vi "Fade In.vi"(7 "Stop Demo":refnum<user-event>, 8 "error in":errorcluster, 10 "VI":refnum<vi>, 11 "Main Subpanel":refnum<vi>) -> (0 "error out":errorcluster)   [LabVIEW 2020]
uses:
  <vilib>/Utility/miscctls.llb/LVRectTypeDef.ctl
  <vilib>/Utility/miscctls.llb/LVPointTypeDef.ctl
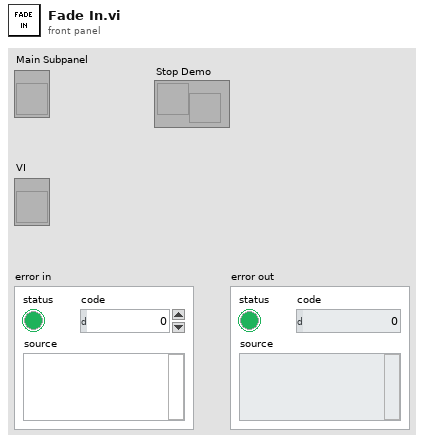
[diagram p1: front panel]
types:
  T1 = typedef "LVPointTypeDef.ctl" = cluster{"Horizontal":i16, "Vertical":i16}
  T2 = enum32{"Invalid", "Standard", "Closed", "Hidden", "Minimized", "Maximized"}
  T3 = typedef "LVRectTypeDef.ctl" = cluster{"Left":i16, "Top":i16, "Right":i16, "Bottom":i16}
  T4 = typedef "LVBoundsTypeDef.ctl" = cluster{"Width":u32, "Height":u32}
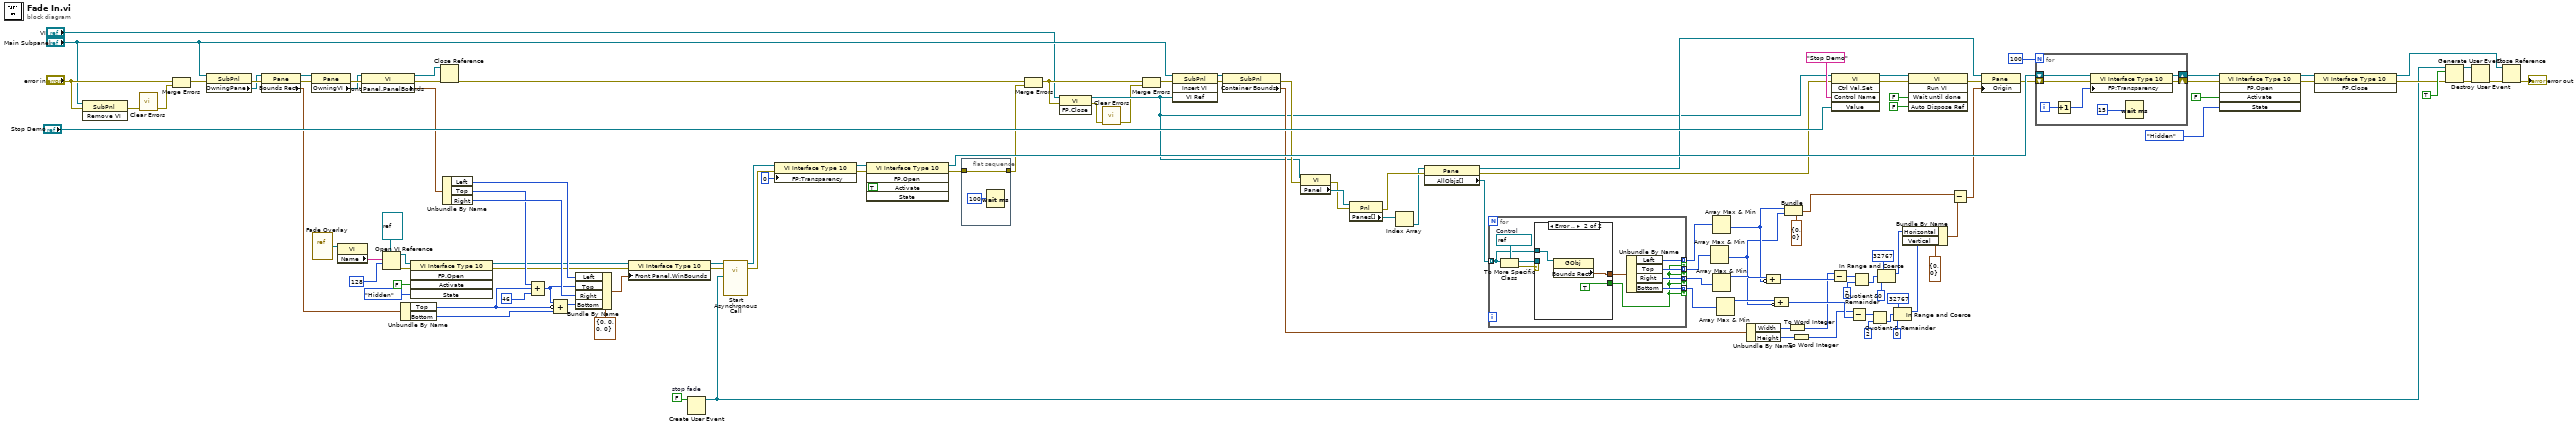
[diagram p0: block diagram]
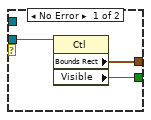
[diagram p2: hidden frame]
diagram:
  w107 = FALSE  # stop fade
  n1 = invoke class="SubPnl" method="Remove VI"(reference="Main Subpanel", error in="error in") -> (error out=w120:errorcluster)  [unwired: 1 in, 2 out]
  n2 = call <vilib>:"Clear Errors.vi"("error in (no error)"=w120) -> ("error out"=w118:errorcluster)  [unwired: 5 in, 1 out]
  n3 = Merge Errors("error in", w118) -> (w82:errorcluster)
  n4 = property class="SubPnl"(reference="Main Subpanel", error in=w82) -> (error out=w90:errorcluster, "OwningPane"=w89:refnum<vi>)  [unwired: 1 out]
  n5 = property class="Pane"(reference=w89, error in=w90) -> (reference out=w87:refnum<vi>, error out=w88:errorcluster, "Bounds Rect"=w80:T3)
  n6 = property class="Pane"(reference=w87, error in=w88) -> (error out=w86:errorcluster, "OwningVI"=w85:refnum<vi>)  [unwired: 1 out]
  n7 = vi-ref "Fade Overlay.vi"() -> (w106:refnum<vi>)
  n8 = property class="VI"(reference=w106) -> ("Name"=w105:string)  [unwired: 1 in, 2 out]
  n9 = property class="VI"(reference=w85, error in=w86) -> (reference out=w83:refnum<vi>, error out=w84:errorcluster, "Front Panel.PanelBounds"=w79:T3)
  n10 = Open VI Reference(type specifier VI Refnum (for type only)=refnum<vi> refnum, vi path=w105, options=128) -> (vi reference=w55:refnum<vi>, error out=w56:errorcluster)  [unwired: 3 in]
  n11 = Unbundle By Name(w80) -> ("Top"=w92:i16, "Bottom"=w93:i16)
  n12 = invoke class="VI Interface Type 10" method="FP.Open"(reference=w55, error in=w56, "Activate"=FALSE ("Activate?"), "State"=T2."Hidden") -> (reference out=w53:refnum<vi>, error out=w54:errorcluster)  [unwired: 1 in, 3 out]
  n13 = Close Reference(reference=w83, error in (no error)=w84) -> (error out=w77:errorcluster)
  n14 = Unbundle By Name(w79) -> ("Left"=w98:i16, "Top"=w96:i16, "Right"=w97:i16)
  n15 = Compound Arithmetic op=ADD(w96, w92, i16 46 ("value")) -> (w95:i16)
  n16 = Compound Arithmetic op=ADD(w95, invert w92, w93) -> (w94:i16)
  n17 = Bundle By Name(cluster=T3 {"Left"=0, "Top"=0, "Right"=0, "Bottom"=0} ("Front Panel Window:Panel Bounds"), "Left"=w98, "Top"=w95, "Right"=w97, "Bottom"=w94) -> (w99:T3)
  n18 = property class="VI Interface Type 10"(reference=w53, error in=w54, "Front Panel.WinBounds"=w99) -> (reference out=w51:refnum<vi>, error out=w52:errorcluster)
  n19 = Create User Event(user event datatype=w107) -> (user event=w65:refnum<user-event>)  [unwired: 1 in, 1 out]
  n20 = call-by-ref "Start Asynchronous Call"(reference=w51, error in=w52, "Stop Fade"=w65) -> (reference out=w101:refnum<vi>, error out=w78:errorcluster)  [unwired: 11 in]
  n21 = property class="VI Interface Type 10"(reference=w101, error in=w78, "FP:Transparency"=u8 0 ("Front Panel Window:Transparency")) -> (reference out=w75:refnum<vi>, error out=w76:errorcluster)
  n22 = invoke class="VI Interface Type 10" method="FP.Open"(reference=w75, error in=w76, "Activate"=TRUE ("Activate?")) -> (reference out=w74:refnum<vi>, error out=w63:errorcluster)  [unwired: 2 in, 3 out]
  n23 = flat-sequence {
    tunnel: [w122] -> w62
    tunnel: w63 -> [w122]
    frame #0 {
      n24 = Wait (ms)(milliseconds to wait=u32 100) -> ()  [unwired: 1 out]
    }
  }
  n25 = Merge Errors(w77, w62) -> (w6:errorcluster)
  n26 = invoke class="VI" method="FP.Close"(reference="VI", error in=w6) -> (reference out=w5:refnum<vi>, error out=w2:errorcluster)  [unwired: 1 in, 1 out]
  n27 = call <vilib>:"Clear Errors.vi"("error in (no error)"=w2) -> ("error out"=w1:errorcluster)  [unwired: 5 in, 1 out]
  n28 = Merge Errors(w6, w1) -> (w3:errorcluster)
  n29 = invoke class="SubPnl" method="Insert VI"(reference="Main Subpanel", error in=w3, "VI Ref"=w5) -> (reference out=w49:refnum<vi>, error out=w50:errorcluster)  [unwired: 1 in, 2 out]
  n30 = property class="SubPnl"(reference=w49, error in=w50) -> (error out=w16:errorcluster, "Container Bounds"=w15:T4)  [unwired: 1 out]
  n31 = property class="VI"(reference=w5, error in=w16) -> (error out=w46:errorcluster, "Panel"=w48:refnum<vi>)  [unwired: 1 out]
  n32 = property class="Pnl"(reference=w48, error in=w46) -> (error out=w45:errorcluster, "Panes[]"=w47:refnum<vi>[])  [unwired: 1 out]
  n33 = Index Array(array=w47) -> (element=w44:refnum<vi>)  [unwired: 1 in]
  n34 = property class="Pane"(reference=w44, error in=w45) -> (reference out=w13:refnum<vi>, error out=w12:errorcluster, "AllObjs[]"=w43:refnum<vi>[])
  n35 = for {
    tunnel: w43 -> [w129] mode=indexing
    tunnel: [w127] -> w42 mode=indexing if=w123
    tunnel: [w126] -> w41 mode=indexing if=w123
    tunnel: [w125] -> w40 mode=indexing if=w123
    tunnel: [w124] -> w39 mode=indexing if=w123
    w131 = refnum<vi> refnum  # Control
    n36 = To More Specific Class(target class=w131, reference=w129) -> (specific class reference=w132:refnum<vi>, error out=w130:errorcluster)  [unwired: 1 in]
    n37 = case shown="Error .." w130 {
      tunnel: w132 -> [w135 _]
      tunnel: w129 -> [_ w138]
      tunnel: [w134 w137] -> w128
      tunnel: [w133 TRUE] -> w123
      frame No Error {
        n38 = property class="Ctl"(reference=w135) -> ("Bounds Rect"=w134:T3, "Visible"=w133:bool)  [unwired: 1 in, 2 out]
      }
      frame Error {
        n39 = property class="GObj"(reference=w138) -> ("Bounds Rect"=w137:T3)  [unwired: 1 in, 2 out]
      }
    }
    n40 = Unbundle By Name(w128) -> ("Left"=w127:i16, "Top"=w126:i16, "Right"=w125:i16, "Bottom"=w124:i16)
  }
  n41 = Array Max & Min(array=w41) -> (min value=w9:i16)  [unwired: 3 out]
  n42 = Array Max & Min(array=w42) -> (min value=w10:i16)  [unwired: 3 out]
  n43 = Array Max & Min(array=w40) -> (max value=w38:i16)  [unwired: 3 out]
  n44 = Array Max & Min(array=w39) -> (max value=w37:i16)  [unwired: 3 out]
  n45 = Unbundle By Name(w15) -> ("Width"=w33:u32, "Height"=w26:u32)
  n46 = Compound Arithmetic op=ADD(w38, invert w10) -> (w34:i16)
  n47 = Compound Arithmetic op=ADD(w37, invert w9) -> (w25:i16)
  n48 = Bundle(cluster=T1 {"Horizontal"=0, "Vertical"=0} ("Origin"), "Horizontal"=w10, "Vertical"=w9) -> (w8:T1)
  n49 = To Word Integer(number=w33) -> (16bit integer=w23:i16)
  n50 = To Word Integer(number=w26) -> (16bit integer=w22:i16)
  n51 = Subtract(x=w23, y=w34) -> (x-y=w32:i16)
  n52 = invoke class="VI" method="Ctrl Val.Set"(reference=w5, error in=w12, "Control Name"="Stop Demo", "Value"="Stop Demo") -> (reference out=w112:refnum<vi>, error out=w116:errorcluster)  [unwired: 1 in, 3 out]
  n53 = Subtract(x=w22, y=w25) -> (x-y=w27:i16)
  n54 = Quotient & Remainder(x=w32, y=i16 2) -> (floor(x/y)=w20:i16)  [unwired: 1 out]
  n55 = Quotient & Remainder(x=w27, y=i16 2) -> (floor(x/y)=w19:i16)  [unwired: 1 out]
  n56 = In Range and Coerce(upper limit=i16 32767, x=w20, lower limit=i16 0) -> (coerced(x)=w29:i16)  [unwired: 1 out]
  n57 = In Range and Coerce(upper limit=i16 32767, x=w19, lower limit=i16 0) -> (coerced(x)=w24:i16)  [unwired: 1 out]
  n58 = Bundle By Name(cluster=T1 {"Horizontal"=0, "Vertical"=0} ("Origin"), "Horizontal"=w29, "Vertical"=w24) -> (w35:T1)
  n59 = invoke class="VI" method="Run VI"(reference=w112, error in=w116, "Wait until done"=FALSE ("Wait Until Done"), "Auto Dispose Ref"=FALSE ("Auto Dispose Reference")) -> (error out=w113:errorcluster)  [unwired: 1 in, 4 out]
  n60 = Subtract(x=w8, y=w35) -> (x-y=w11:T1)
  n61 = property class="Pane"(reference=w13, error in=w113, "Origin"=w11) -> (error out=w14:errorcluster)  [unwired: 1 out]
  n62 = for {
    N: 100 -> [_]
    shift-right: [w142] -> w60
    shift-left: w74 -> [w143]
    shift-right: [w144] -> w69
    shift-left: w14 -> [w145]
    i -> [w140]
    n63 = Increment(x=w140) -> (x+1=w139:i32)
    n64 = property class="VI Interface Type 10"(reference=w143, error in=w145, "FP:Transparency"=w139) -> (reference out=w142:refnum<vi>, error out=w144:errorcluster)
    n65 = Wait (ms)(milliseconds to wait=u32 15) -> ()  [unwired: 1 out]
  }
  n66 = invoke class="VI Interface Type 10" method="FP.Open"(reference=w60, error in=w69, "Activate"=FALSE ("Activate?"), "State"=T2."Hidden") -> (reference out=w59:refnum<vi>, error out=w61:errorcluster)  [unwired: 1 in, 3 out]
  n67 = invoke class="VI Interface Type 10" method="FP.Close"(reference=w59, error in=w61) -> (reference out=w66:refnum<vi>, error out=w68:errorcluster)  [unwired: 1 in, 1 out]
  n68 = Generate User Event(user event=w65, event data cluster=TRUE ("event data"), error in=w68) -> (user event out=w71:refnum<user-event>, error out=w72:errorcluster)  [unwired: 1 in]
  n69 = Destroy User Event(user event=w71, error in=w72) -> (error out=w70:errorcluster)
  n70 = Close Reference(reference=w66, error in (no error)=w70) -> (error out=→"error out":errorcluster)
